vi "ALS control remote.vi"(11 "Connection type":enum16{"Local", "Remote"}(ring)=enum."Remote") -> ()   [LabVIEW 2017]
panel:
  in  "Stop Button":bool
  in  "ChemStation Name":string="hpcore7544"
  in  "Method name":string="DropPrep.M"
  out "DDE control":i8
  # "Only use this VI on the PC where ChemStation is installed."
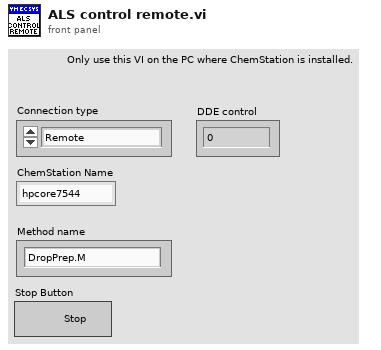
[diagram p1: front panel]
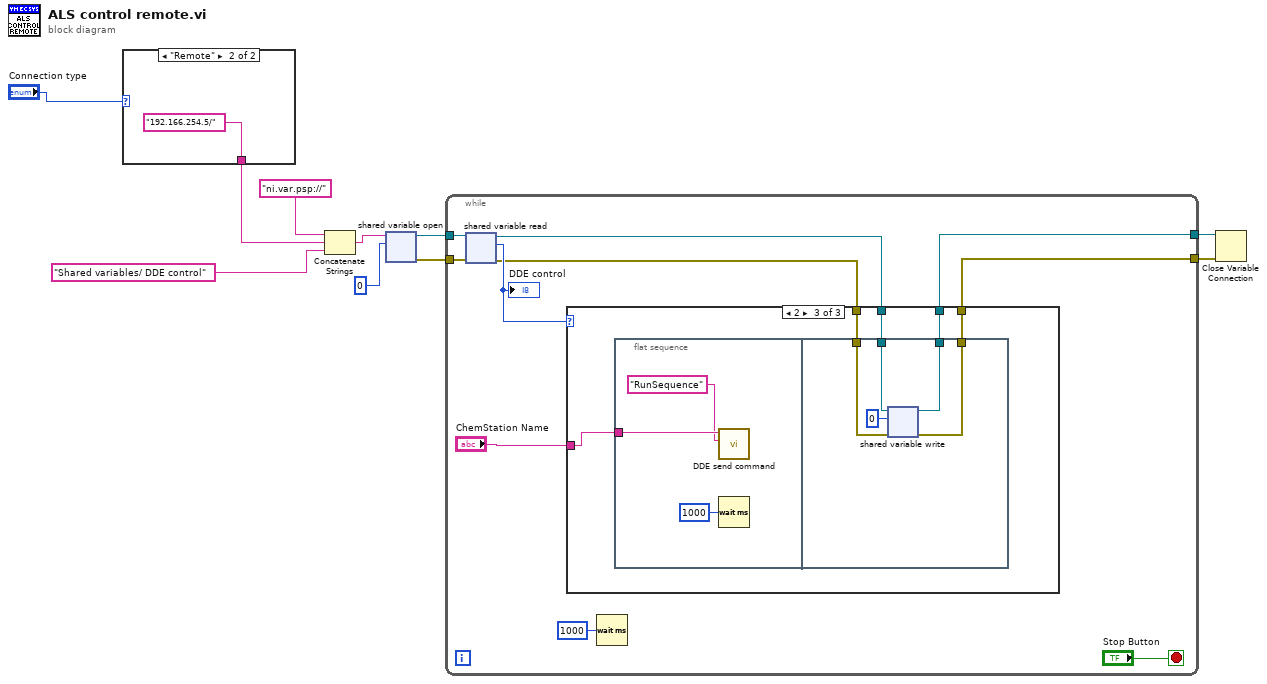
[diagram p0: block diagram]
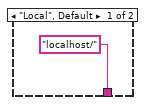
[diagram p2: hidden frame]
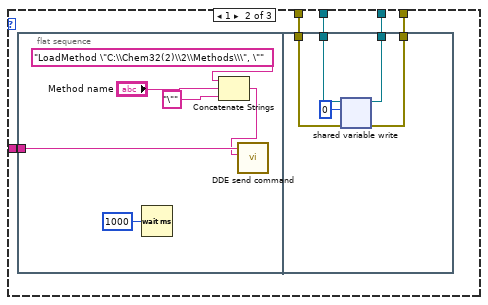
[diagram p4: hidden frame]
diagram:
  n1 = case shown="\"Remote\"" "Connection type" {
    tunnel: ["localhost/" "192.166.254.5/"] -> w7
    frame "Local", Default {
    }
    frame "Remote" {
    }
  }
  n2 = Concatenate Strings("ni.var.psp://" ("string"), w7, "Shared variables/ DDE control") -> (w6:string)
  n3 = shared-variable-open(w6, i8 0) -> (w4:refnum<k21>, w3:errorcluster)  [unwired: 2 in]
  n4 = while {
    tunnel: w4 -> [w22]
    tunnel: w3 -> [w21]
    tunnel: [w15] -> w2
    tunnel: [w14] -> w1
    stop <- "Stop Button" stop-if-true
    n5 = shared-variable-read(w22, w21) -> (w17:refnum<k21>, w18:errorcluster, w20:i8)  [unwired: 1 out]
    "DDE control" <- w20
    n6 = case shown="2" w20 {
      tunnel: w18 -> [w23 w27 w43]
      tunnel: w17 -> [w24 w28 w44]
      tunnel: "ChemStation Name" -> [_ w29 w45]
      tunnel: [w24 w26 w42] -> w14
      tunnel: [w23 w25 w41] -> w15
      frame 0, Default {
      }
      frame 1 {
        n7 = flat-sequence {
          tunnel: w29 -> [w32]
          tunnel: w28 -> [w40]
          tunnel: w27 -> [w39]
          tunnel: [w37] -> w26
          tunnel: [w36] -> w25
          frame #0 {
            n8 = Wait (ms)(milliseconds to wait=u32 1000) -> ()  [unwired: 1 out]
            n9 = Concatenate Strings("LoadMethod \"C:\\Chem32(2)\\2\\Methods\\\", \"", "Method name", "\"" ("string")) -> (w31:string)
            n10 = call "DDE send command.vi"("Command"=w31, "ChemStation Name"=w32) -> ()  [unwired: 10 in]
          }
          frame #1 {
            n11 = shared-variable-write(w40, w39, i8 0 ("data in")) -> (w37:refnum<k21>, w36:errorcluster)
          }
        }
      }
      frame 2 {
        n12 = flat-sequence {
          tunnel: w45 -> [w48]
          tunnel: w44 -> [w53]
          tunnel: w43 -> [w52]
          tunnel: [w50] -> w42
          tunnel: [w49] -> w41
          frame #0 {
            n13 = call "DDE send command.vi"("Command"="RunSequence", "ChemStation Name"=w48) -> ()  [unwired: 10 in]
            n14 = Wait (ms)(milliseconds to wait=u32 1000) -> ()  [unwired: 1 out]
          }
          frame #1 {
            n15 = shared-variable-write(w53, w52, i8 0 ("data in")) -> (w50:refnum<k21>, w49:errorcluster)
          }
        }
      }
    }
    n16 = Wait (ms)(milliseconds to wait=u32 1000) -> ()  [unwired: 1 out]
  }
  n17 = Close Variable Connection(8:w2, 11:w1) -> ()  [unwired: 1 out]
